vi "Setup Refs.vi"(8 "error in (no error)":errorcluster, 10 "Device Reference in":T5 format="%.0x", 11 "RT Data In":T1={" Inputs"={"Vals"=[], "When"=[], "Data Refs"=[], "Session"=""}, "Outputs"={"Vals"=[], "When"=[], "Data Refs"=[], "Session"=""}, "Internal Iteration"=-2, "Device Error"={"status"=FALSE, "code"=0, "source"=""}} {"Outputs"."Data Refs" format="%.0x"; "Inputs"."Data Refs" format="%.0x"}) -> (0 "error out":errorcluster, 3 "RT Data Out":T1={" Inputs"={"Vals"=[], "When"=[], "Data Refs"=[], "Session"=""}, "Outputs"={"Vals"=[], "When"=[], "Data Refs"=[], "Session"=""}, "Internal Iteration"=-2, "Device Error"={"status"=FALSE, "code"=0, "source"=""}} {"Outputs"."Data Refs" format="%.0x"; "Inputs"."Data Refs" format="%.0x"}, 5 "Hz":u32)   [LabVIEW 2010, in "XNET Reflective Memory Custom Device.lvlib"]
uses:
  XNET Reflective Memory Custom Device.lvlib
  <vilib>/NI VeriStand/Custom Device API/Custom Device Item Ref.ctl
  RT DATA.ctl
  Single Category.ctl
  BeforeAfter.ctl
  <vilib>/NI VeriStand/Custom Device API/Data Reference.ctl
  <vilib>/NI VeriStand/Custom Device API/Custom Device Channel Type.ctl
  <vilib>/NI VeriStand/Custom Device API/Data Access Type.ctl
  <vilib>/xnet/xnet.llb/XNET Mode.ctl
  Global.vi
  <vilib>/NI VeriStand/Custom Device API/Get Item Property (String).vi
  <vilib>/xnet/xnet.llb/XNET String To IO Name (Interface).vi
  <vilib>/xnet/xnet.llb/XNET Create Session (Generic).vi
  <vilib>/NI VeriStand/Custom Device API/Get Item Property (U16).vi
  <vilib>/NI Veristand/Custom Device API/Custom Device API.lvlib
  Program Files/National Instruments/LabVIEW 2010/resource/objmgr/xnet.rc
  <vilib>/xnet/xnet.llb/XNET String To IO Name (Cluster).vi
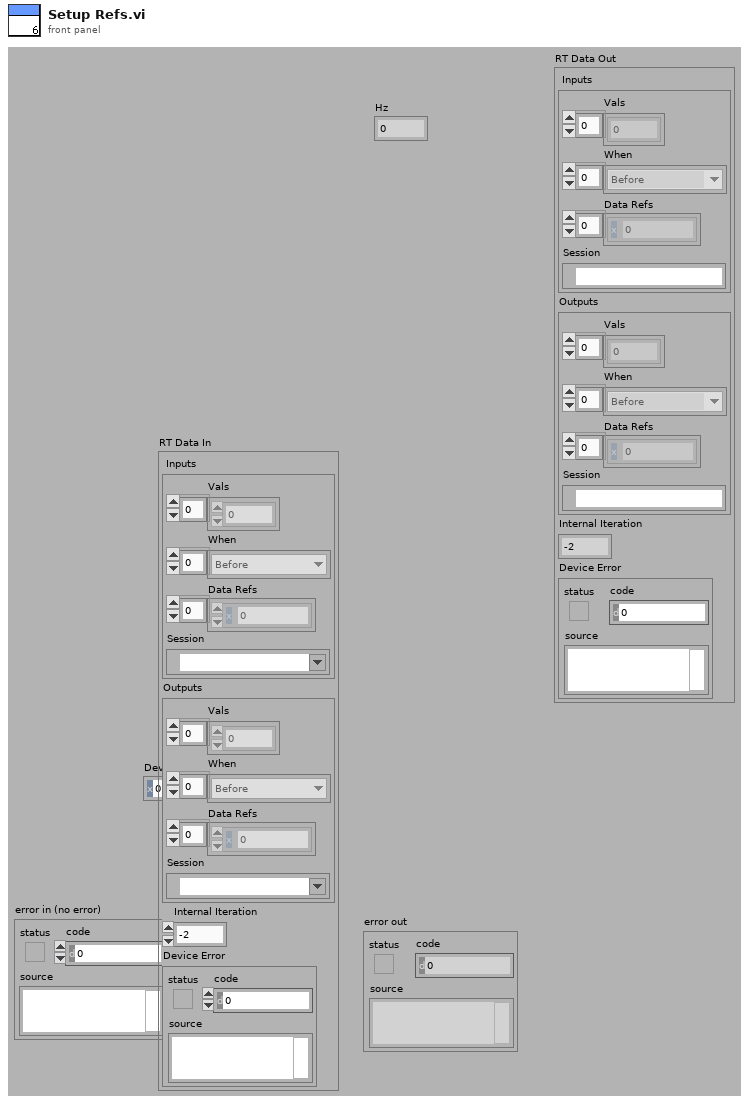
[diagram p1: front panel]
types:
  T1 = typedef "XNET Reflective Memory Custom Device.lvlib/RT DATA.ctl" = cluster{" Inputs":T2, "Outputs":T2, "Internal Iteration":i32, "Device Error":errorcluster}
  T2 = typedef "XNET Reflective Memory Custom Device.lvlib/Single Category.ctl" = cluster{"Vals":dbl[], "When":T3[], "Data Refs":T4[], "Session":refnum<k21>}
  T3 = typedef "XNET Reflective Memory Custom Device.lvlib/BeforeAfter.ctl" = enum16{"Before", "After"}
  T4 = typedef "Custom Device API.lvlib/Data Reference.ctl" = i32
  T5 = typedef "Custom Device API.lvlib/Custom Device Item Ref.ctl" = u64
  T6 = typedef "XNET Mode.ctl" = u32
  T7 = typedef "Custom Device API.lvlib/Data Access Type.ctl" = enum16{"Read", "Write"}
  T8 = typedef "Custom Device API.lvlib/Custom Device Channel Type.ctl" = enum16{"Input", "Output"}
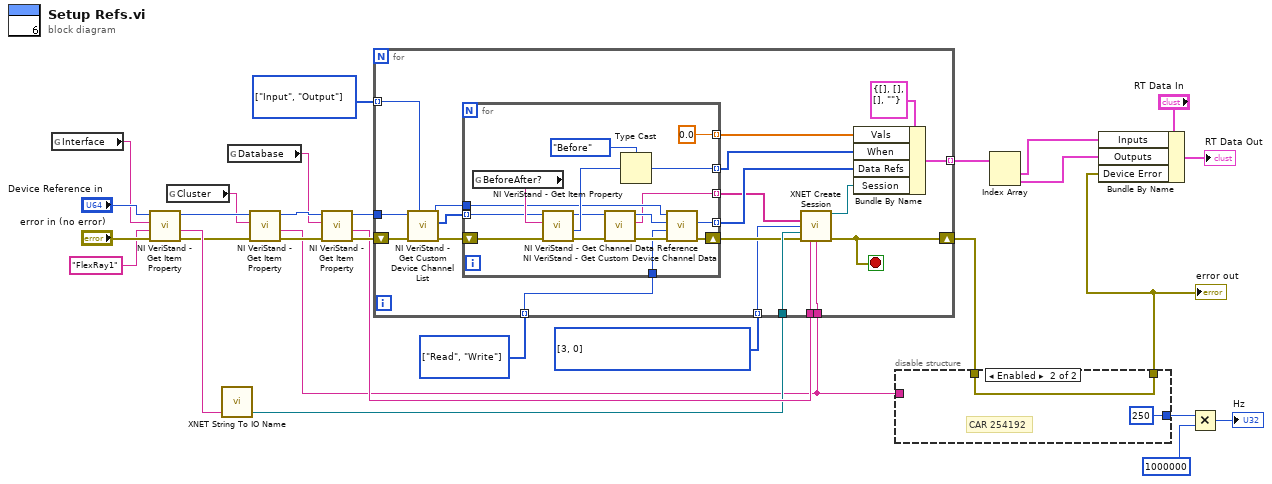
[diagram p0: block diagram]
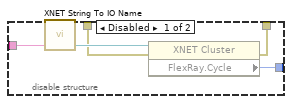
[diagram p2: hidden frame]
diagram:
  w4 = T6[] [3, 0] items=["Signal Input Single-point", "Signal Input Waveform", "Signal Input XY", "Signal Output Single-point", "Signal Output Waveform", "Signal Output XY", "Frame Input Stream", "Frame Input Queued", "Frame Input Single-point", "Frame Output Stream", "Frame Output Queued", "Frame Output Single-point"]
  w5 = T7[] [enum."Read", enum."Write"] items=["Read", "Write"]
  w29 = T8[] [enum."Input", enum."Output"] items=["Input", "Output"]
  n1 = global read "Global.vi" "Interface"() -> (w24:string)
  n2 = call-poly <vilib>:"NI VeriStand - Get Item Property.vi"("error in (no error)"="error in (no error)", "Default Value"="FlexRay1", "Property Name"=w24, "Item Ref in"="Device Reference in") -> ("error out"=w21:errorcluster, "Value"=w22:string, "Item Ref out"=w20:T5)  [unwired: 4 in, 1 out]
  n3 = global read "Global.vi" "Cluster"() -> (w15:string)
  n4 = call-poly <vilib>:"XNET String To IO Name.vi"("string"=w22) -> ("XNET Interface"=w12:refnum<k21>)  [unwired: 4 in]
  n5 = global read "Global.vi" "Database"() -> (w14:string)
  n6 = call-poly <vilib>:"NI VeriStand - Get Item Property.vi"("error in (no error)"=w21, "Property Name"=w15, "Item Ref in"=w20) -> ("error out"=w16:errorcluster, "Value"=w9:string, "Item Ref out"=w19:T5)  [unwired: 5 in, 1 out]
  n7 = call-poly <vilib>:"NI VeriStand - Get Item Property.vi"("error in (no error)"=w16, "Property Name"=w14, "Item Ref in"=w19) -> ("error out"=w17:errorcluster, "Value"=w13:string, "Item Ref out"=w18:T5)  [unwired: 5 in, 1 out]
  n8 = for {
    tunnel: w29 -> [w45] mode=indexing
    shift-right: [w31] -> w8
    shift-left: w17 -> [w49]
    tunnel: w18 -> [w48]
    tunnel: w12 -> [w44]
    tunnel: w13 -> [w43]
    tunnel: w9 -> [w42]
    tunnel: w5 -> [w41] mode=indexing
    tunnel: w4 -> [w38] mode=indexing
    tunnel: [w32] -> w3 mode=indexing
    stop <- w31 stop-if-true
    n9 = call <vilib>:"NI VeriStand - Get Custom Device Channel List.vi"("Channel Type"=w45, "error in (no error)"=w49, "Device Ref in"=w48) -> ("error out"=w46:errorcluster, "Specified Channel Ref List"=w47:T5[], "Device Ref out"=w40:T5)  [unwired: 6 out]
    n10 = for {
      tunnel: w47 -> [w61] mode=indexing
      shift-right: [w57] -> w39
      shift-left: w46 -> [w65]
      tunnel: w41 -> [w56]
      tunnel: w40 -> [w55]
      tunnel: [w53] -> w34 mode=indexing
      tunnel: [w52] -> w30 mode=indexing
      tunnel: [w51] -> w33 mode=indexing
      tunnel: [0.0] -> w36 mode=indexing
      n11 = global read "Global.vi" "BeforeAfter?"() -> (w64:string)
      n12 = call-poly <vilib>:"NI VeriStand - Get Item Property.vi"("error in (no error)"=w65, "Property Name"=w64, "Item Ref in"=w61) -> ("error out"=w60:errorcluster, "Value"=w63:u16, "Item Ref out"=w59:T5)  [unwired: 5 in, 1 out]
      n13 = call <vilib>:"NI VeriStand - Get Custom Device Channel Data.vi"("error in (no error)"=w60, "Channel Ref in"=w59) -> ("error out"=w58:errorcluster, "Channel Name"=w52:string, "Channel Ref out"=w54:T5)  [unwired: 4 in, 3 out]
      n14 = Type Cast(type=BeforeAfter."Before" ("BeforeAfter?"), x=w63) -> (*(type *) &x=w51:T3)
      n15 = call <vilib>:"NI VeriStand - Get Channel Data Reference.vi"("error in (no error)"=w58, "Access"=w56, "Channel Ref in"=w54, "Device Ref in"=w55) -> ("error out"=w57:errorcluster, "Channel Data Reference"=w53:T4)  [unwired: 5 in, 1 out]
    }
    n16 = call-poly <vilib>:"XNET Create Session.vi"("list (empty)"=w30, "mode"=w38, "interface"=w44, "error in (no error)"=w39, "database (:memory:)"=w43, "cluster (empty)"=w42) -> ("session out"=w35:refnum<k21>, "error out"=w31:errorcluster)  [unwired: 8 in]
    n17 = Bundle By Name(cluster=T2 {"Vals"=[], "When"=[], "Data Refs"=[], "Session"=""}, "Vals"=w36, "When"=w33, "Data Refs"=w34, "Session"=w35) -> (w32:T2)
  }
  n18 = disable-structure shown="Enabled" {
    disable-tunnel: [w69 u32 250 ("FlexRay.Cycle")] -> w11
    disable-tunnel: w9 -> [w68 _]
    disable-tunnel: w8 -> [w67 w71]
    disable-tunnel: [w66 w71] -> w6
    frame Disabled {
      n19 = call-poly <vilib>:"XNET String To IO Name.vi"("string"=w68) -> ("XNET Cluster"=w70:refnum<k21>)  [unwired: 4 in]
      n20 = property class="XNET Cluster"(reference=w70, error in=w67) -> (error out=w66:errorcluster, "FlexRay.Cycle"=w69:u32)  [unwired: 1 out]
    }
    frame Enabled {
      # "CAR 254192"
    }
  }
  "error out" <- w6
  n21 = Index Array(array=w3) -> (element #1=w2:T2, element #2=w1:T2)  [unwired: 2 in]
  n22 = Bundle By Name(cluster="RT Data In", "Inputs"=w2, "Outputs"=w1, "Device Error"=w6) -> (→"RT Data Out":T1)
  n23 = Multiply(x=w11, y=u32 1000000) -> (x*y=→"Hz":u32)
